vi "CreateSelfReference.vi"(8 "error in (no error)":errorcluster, 11 "Camera.Simulated":refnum<class "Camera.Simulated.lvclass">) -> (0 "error out":errorcluster, 3 "Camera.Simulated out":refnum<class "Camera.Simulated.lvclass">)   [LabVIEW 2013, in "Camera.Simulated.lvclass"]
doc: "JKI State Machine Objects (SMO) 1.0.0.5\nJKI - JKI\nCopyright (c) 2016, JKI"
uses:
  Camera.Simulated.lvclass
  Camera/Camera.lvclass
panel:
  # "For instructions on how to use the JKI State Machine Objects, examples and video tutorials, visit:\nhttp://jki.net/state-machine-objects/\n\nJKI State Machine Objects™\nhttp://jki.net/state-machine-objects/\nCopyright (C) 2005-2015, JKI <info@jki.net>\nALL RIGHTS RESERVED"
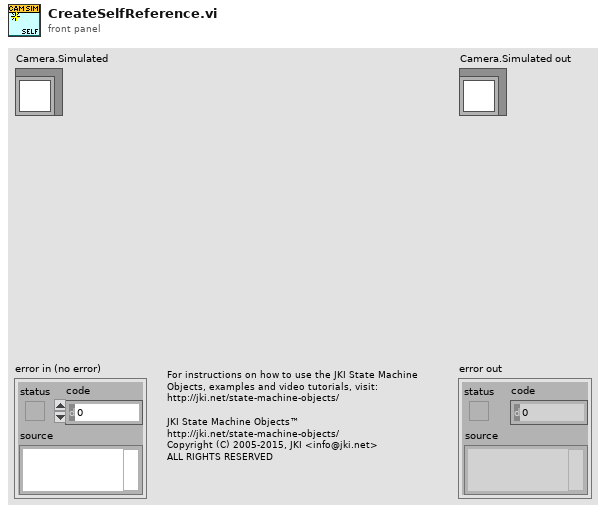
[diagram p1: front panel]
types:
  T1 = typedef "Camera.Simulated.lvclass/PrivateData--Ref.ctl" = refnum<data-value>
  T2 = typedef "Camera.Simulated.lvclass/PrivateData--Cluster.ctl" = cluster{"Dependencies":T3, "Configuration":T4}
  T3 = typedef "Camera.Simulated.lvclass/Dependencies--Cluster.ctl" = cluster{"CircularBuffer.ImageData":refnum<class "CircularBuffer.ImageData.lvclass">}
  T4 = typedef "Camera.Simulated.lvclass/Configuration--CLuster.ctl" = cluster{"Simulated Images Folder":path, "filetype":string}
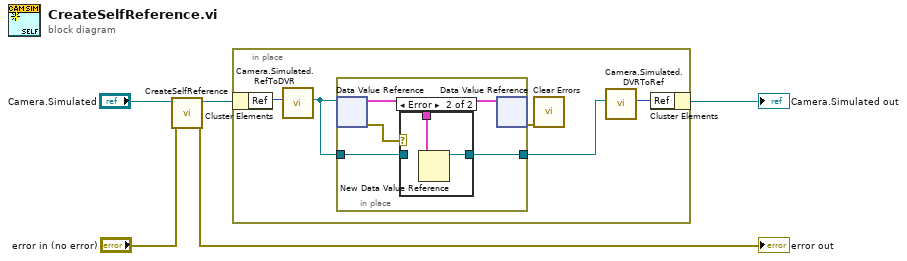
[diagram p0: block diagram]
diagram:
  n1 = call-parent "CreateSelfReference.vi"("error in (no error)"="error in (no error)", "Camera"="Camera.Simulated") -> ("error out"=→"error out":errorcluster, "Camera out"=w4:refnum<class "Camera.Simulated.lvclass">)  [unwired: 8 in]
  n2 = in-place {
    n3 = in-place-cluster #1(w4) -> ("Ref"=w7:u32)
    n4 = call "Camera.Simulated.RefToDVR.vi"("Ref"=w7) -> ("Ref"=w6:T1)  [unwired: 10 in]
    n5 = in-place {
      in-place-border: [w14] -> w9
      in-place-border: w6 -> [w11]
      n6 = in-place-dvr #2(w6) -> (w13:T2, w12:errorcluster)
      n7 = case shown="Error" w12 {
        tunnel: [w15 w17] -> w14
        tunnel: w13 -> [_ w16]
        tunnel: w11 -> [w15 _]
        frame No Error {
        }
        frame Error {
          n8 = New Data Value Reference(data value=w16) -> (data value reference=w17:refnum<data-value>)  [unwired: 1 in, 1 out]
        }
      }
      n9 = in-place-dvr #2(w13) -> (w10:errorcluster)  [unwired: 1 out]
    }
    n10 = call <vilib>:"Clear Errors.vi"("error in (no error)"=w10) -> ()  [unwired: 5 in, 2 out]
    n11 = call "Camera.Simulated.DVRToRef.vi"("Ref"=w9) -> ("Ref"=w8:u32)  [unwired: 10 in]
    n12 = in-place-cluster #1("Ref"=w8) -> (→"Camera.Simulated out":refnum<class "Camera.Simulated.lvclass">)
  }
